vi "Errorbar0003.vi"   [LabVIEW 2013]
uses:
  <vilib>/Heliosphere Research LLC/Advanced Plotting Toolkit/api_core/NewPlotType.ctl
  ModeType.ctl
  ErrorCodes.ctl
  <vilib>/Heliosphere Research LLC/Advanced Plotting Toolkit/Advanced Plotting Toolkit.lvlib
types:
  T1 = typedef "ErrorCodes.ctl" = u32
  T2 = typedef "ModeType.ctl" = enum16{"Normal", "Expected Failure", "Skipped", "Broken"}
  T3 = typedef "Advanced Plotting Toolkit.lvlib/NewPlotType.ctl" = enum16{"Rectangular Axes", "Polar Axes"}
  T4 = typedef "Advanced Plotting Toolkit.lvlib/PlotID.ctl" = i32
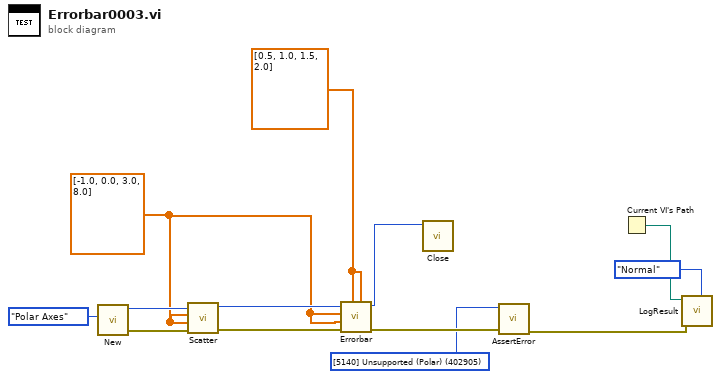
[diagram p0: block diagram]
diagram:
  w1 = T1 402905 items=["[5120] Invalid ID"=402902, "[5110] Failed to Init"=402900, "[5111] Unknown Error"=402901, "[5130] Save - Bad File Extension"=402403, "[5131] Save - General Error"=402904, "[5140] Unsupported (Polar)"=402905, "[5141] Unsupported (Logscale)"=402906, "[5142] Coordinates Not Regular"=402907] ("Expected Error")
  w7 = dbl[] [0.5, 1.0, 1.5, 2.0] ("X Errors")
  w8 = dbl[] [-1.0, 0.0, 3.0, 8.0] ("X Data")
  n1 = call <vilib>:"New.vi"("Plot Type"=NewPlotType."Polar Axes") -> ("error out"=w9:errorcluster, "Plot ID"=w12:T4)  [unwired: 9 in]
  n2 = call <vilib>:"Scatter.vi"("error in (no error)"=w9, "Y Data"=w8, "X Data"=w8, "Plot ID"=w12) -> ("error out"=w10:errorcluster, "Plot ID Out"=w11:T4)  [unwired: 6 in]
  n3 = call <vilib>:"Errorbar.vi"("Y Errors"=w7, "X Errors"=w7, "error in (no error)"=w10, "Y Data"=w8, "X Data"=w8, "Plot ID"=w11) -> ("error out"=w4:errorcluster, "Plot ID out"=w5:T4)  [unwired: 4 in]
  n4 = call <vilib>:"Close.vi"("Plot ID"=w5) -> ()  [unwired: 10 in, 1 out]
  n5 = call "AssertError.vi"("error in (no error)"=w4, "Expected Error"=w1) -> ("error out"=w3:errorcluster)  [unwired: 9 in]
  n6 = Current VI's Path() -> (path=w13:path)
  n7 = call "LogResult.vi"("Mode"=ModeType."Normal", "Test Result"=w3, "VI Path"=w13) -> ()  [unwired: 9 in]
